vi "RegWrite UnitTest.vi"() -> ()   [LabVIEW 2018]
uses:
  Downloads/MIPI RFFE API/Controls/RFFE Commands Type Def.ctl
  Downloads/MIPI RFFE API/Controls/Write Data Strict Type Def.ctl
  Command/RFFE Command.lvclass
  RegWrite/RFFE RegWrite Command.lvclass
  C:/Users/semoore/Projects/mipi-rffe-labview-oop/Command/RFFE Command.lvclass
panel:
  out "arrays same size?":bool
  out "data equal?":bool
  out "error in (no error) 2":errorcluster
  in  "error in (no error)":errorcluster
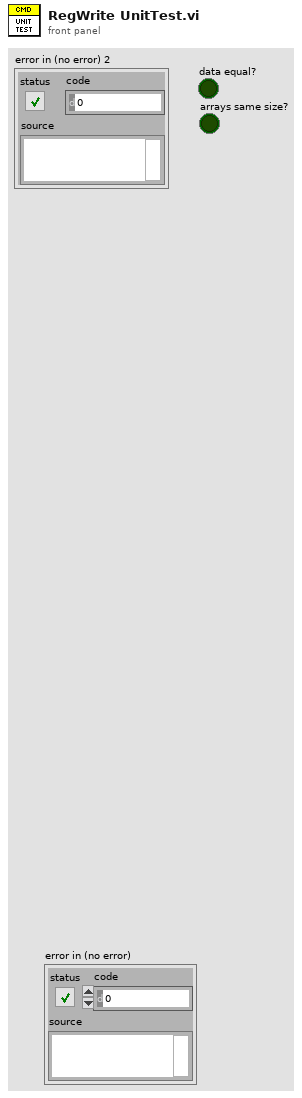
[diagram p1: front panel]
types:
  T1 = typedef "Write Data Strict Type Def.ctl" = cluster{"slave address":u8, "register address":u16, "register data (write)":u8[], "byte count":u8}
  T2 = typedef "RFFE Commands Type Def.ctl" = enum16{"Reg0Write", "RegWrite", "RegRead", "RegReadHR", "RegWriteExt", "RegReadExt", "RegReadExtHR", "RegWriteExtLong", "RegReadExtLong", "RegReadExtLongHR"}
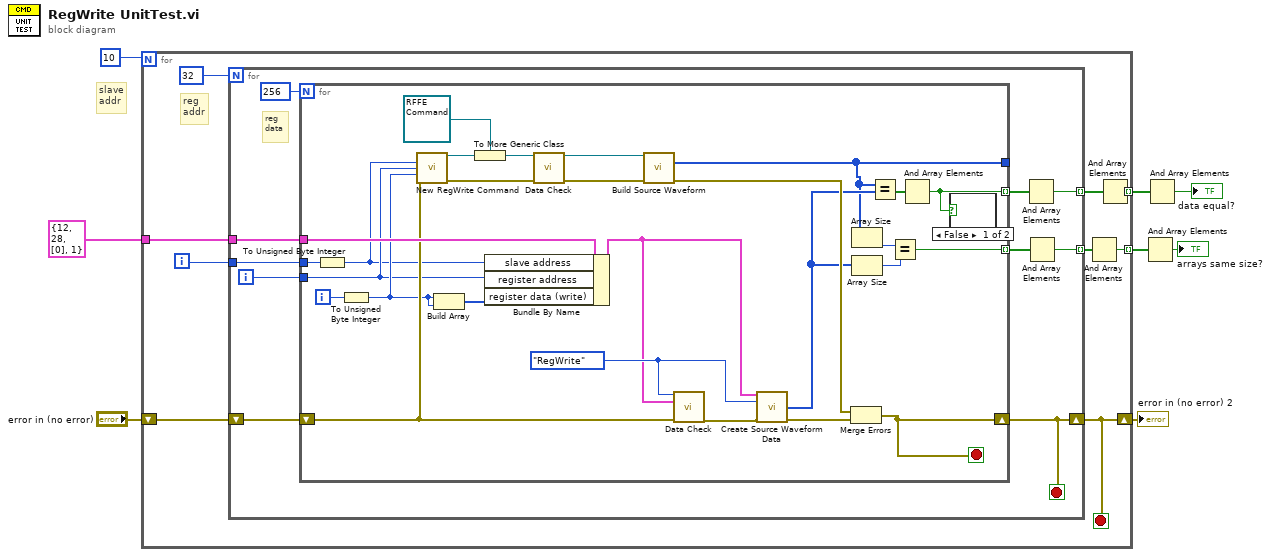
[diagram p0: block diagram]
diagram:
  # "slave\naddr"
  n1 = for {
    N: 10 -> [_]
    tunnel: T1 {"slave address"=12, "register address"=28, "register data (write)"=[0], "byte count"=1} ("Register Data") -> [w16]
    shift-right: [w13] -> w5
    shift-left: "error in (no error)" -> [w17]
    tunnel: [w11] -> w4 mode=indexing
    tunnel: [w9] -> w2 mode=indexing
    i -> [w15]
    stop <- w13 stop-if-true
    # "reg\naddr"
    n2 = for {
      N: 32 -> [_]
      tunnel: w16 -> [w26]
      tunnel: w15 -> [w23]
      shift-right: [w22] -> w13
      shift-left: w17 -> [w27]
      tunnel: [w20] -> w12 mode=indexing
      tunnel: [w18] -> w10 mode=indexing
      i -> [w24]
      stop <- w22 stop-if-true
      # "reg\ndata"
      n3 = for {
        N: 256 -> [_]
        tunnel: w26 -> [w52]
        tunnel: [w37] -> _
        tunnel: w24 -> [w30]
        tunnel: w23 -> [w40]
        shift-right: [w44] -> w22
        shift-left: w27 -> [w41]
        tunnel: [w34] -> w21 mode=indexing
        tunnel: [w28] -> w19 mode=indexing
        i -> [w39]
        stop <- w44 stop-if-true
        w54 = RFFE_Commands_Type_Def."RegWrite" ("RFFE command")
        n4 = To Unsigned Byte Integer(number=w40) -> (unsigned 8bit integer=w29:u8)
        n5 = To Unsigned Byte Integer(number=w39) -> (unsigned 8bit integer=w31:u8)
        n6 = call "New RegWrite Command.vi"("Slave Address"=w29, "Register Address"=w30, "Register Data"=w31, "error in (no error)"=w41) -> ("RFFE RegWrite Command out"=w48:refnum<class "RFFE RegWrite Command.lvclass">, "error out"=w49:errorcluster)  [unwired: 10 in]
        n7 = Build Array(w31, w31) -> (w46:u8[])
        n8 = To More Generic Class(target class=refnum<class "RFFE Command.lvclass"> refnum ("RFFE Commands.lvlib:RFFE Command.lvclass"), reference=w48) -> (generic class reference=w33:refnum<class "RFFE Command.lvclass">)
        n9 = Bundle By Name(cluster=w52, "slave address"=w29, "register address"=w30, "register data (write)"=w46) -> (w51:T1)
        n10 = call-dynamic "Data Check.vi"("RFFE Command in"=w33, "error in (no error)"=w49) -> ("RFFE Command out"=w47:refnum<class "RFFE Command.lvclass">, "error out"=w50:errorcluster)  [unwired: 12 in]
        n11 = call-dynamic "Build Source Waveform.vi"("RFFE Command in"=w47, "error in (no error)"=w50) -> ("Source Waveform"=w37:u32[], "error out"=w43:errorcluster)  [unwired: 11 in, 1 out]
        n12 = call "Data Check.vi"("RFFE command"=w54, "Register Data"=w51, "error in"=w41) -> ("error out"=w53:errorcluster)  [unwired: 12 in]
        n13 = call "Create Source Waveform Data.vi"("Register Data"=w51, "RFFE command"=w54, "error in"=w53) -> ("RFFEWrite source waveform data array"=w38:u32[], "error out"=w45:errorcluster)  [unwired: 10 in, 1 out]
        n14 = Merge Errors(w43, w45) -> (w44:errorcluster)
        n15 = Array Size(array=w37) -> (size(s)=w36:i32)
        n16 = Array Size(array=w38) -> (size(s)=w35:i32)
        n17 = Equal?(x=w37, y=w38) -> (x = y?=w42:bool[])
        n18 = Equal?(x=w36, y=w35) -> (x = y?=w28:bool)
        n19 = And Array Elements(Boolean array=w42) -> (logical AND=w34:bool)
        n20 = case shown="False" w34 {
          frame False {
          }
          frame True {
          }
        }
      }
      n21 = And Array Elements(Boolean array=w21) -> (logical AND=w20:bool)
      n22 = And Array Elements(Boolean array=w19) -> (logical AND=w18:bool)
    }
    n23 = And Array Elements(Boolean array=w10) -> (logical AND=w9:bool)
    n24 = And Array Elements(Boolean array=w12) -> (logical AND=w11:bool)
  }
  "error in (no error) 2" <- w5
  n25 = And Array Elements(Boolean array=w2) -> (logical AND=→"arrays same size?":bool)
  n26 = And Array Elements(Boolean array=w4) -> (logical AND=→"data equal?":bool)
